vi "ProcessingFrame.vi"(8 "error in (no error)":errorcluster, 11 "navX - Base in":refnum<class "navX - Interface.lvclass">) -> (0 "error out":errorcluster, 3 "navX - Base out":refnum<class "navX - Interface.lvclass">)   [LabVIEW 2015, in "navX Library v3.lvlib" / "navX - Interface.lvclass"]
uses:
  navX - Interface.lvclass
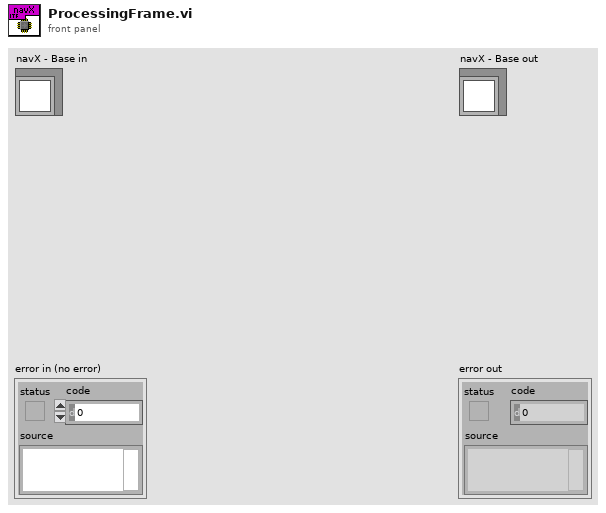
[diagram p1: front panel]
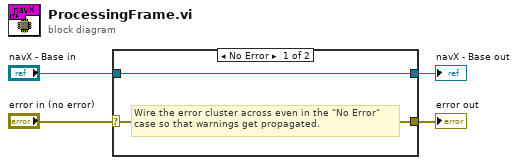
[diagram p0: block diagram]
diagram:
  n1 = case shown="No Error" "error in (no error)" {
    selector: "error in (no error)" -> [w5 w8]
    tunnel: [w5 w8] -> w4
    tunnel: [w6 w7] -> w2
    tunnel: "navX - Base in" -> [w6 w7]
    frame No Error {
      # "Wire the error cluster across even in the \"No Error\"\ncase so that warnings get propagated."
    }
    frame Error {
    }
  }
  "error out" <- w4
  "navX - Base out" <- w2
